vi "34970 Preset Instrument.vi"(8 "error in (no error)":errorcluster, 11 "VISA session":refnum<visa-resource-name>) -> (0 "error out":errorcluster, 3 "dup VISA session":refnum<visa-resource-name>)   [LabVIEW 2020]
doc: "Sends configuration PRESet command to instrument. See p161 34970 User MAnual.\nW. Gilbert, University of Minnesota Physics, 8/6/2004\nwgilbert@physics.umn.edu"
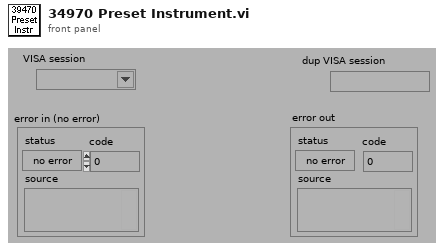
[diagram p1: front panel]
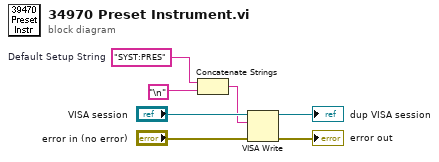
[diagram p0: block diagram]
diagram:
  w3 = "SYST:PRES"  # Default Setup String
  n1 = Concatenate Strings(w3, "\n") -> (w2:string)
  n2 = VISA Write(VISA resource name="VISA session", write buffer=w2, error in (no error)="error in (no error)") -> (VISA resource name out=→"dup VISA session":refnum<visa-resource-name>, error out=→"error out":errorcluster)  [unwired: 1 out]
